vi "MyG#G3SubTempl_GetAttributesToModify.vi"(0 "reference in":refnum<class "MyG#G3SubTempl.lvclass">, 3 "timeout in ms (-1)":i32=-1, 5 "error in (no error)":errorcluster) -> (14 "reference out":refnum<class "MyG#G3SubTempl.lvclass">, 15 "attributes ref":T3, 16 "attributes":T1, 17 "timeout":bool, 19 "error out":errorcluster)   [LabVIEW 2020, in "MyG#G3SubTempl.lvclass"]
doc: "This VI returns the class attributes associated with the object reference and places a lock on the object. If reference is wired, the class attributes of this class (or sub class) will be returned else the class attributes will default to the class.\n\nIf the object is currently locked for modification by another method, 'Timeout' specifies how long the VI should wait to receive access to the object. The default value waits until the object becomes available.\n\nYou must use this class SetModifiedClassAttributes VI to set the object's data and release the lock."
uses:
  MyG#G3SubTempl.lvclass
  C:/Program Files (x86)/National Instruments/LabVIEW 2020/examples/AddQ/G#/CreateDestroy/MyG#G3Templ_class/MyG#G3Templ.lvclass
  ObjectAttributesRef.ctl
  protected/ObjectAttributes.ctl
  MyG#G3Templ_class/protected/ObjectAttributes.ctl
  MyG#G3SubTempl.lvclass/MyG#G3SubTempl.ctl
  MyG#G3Templ_class/MyG#G3Templ.lvclass
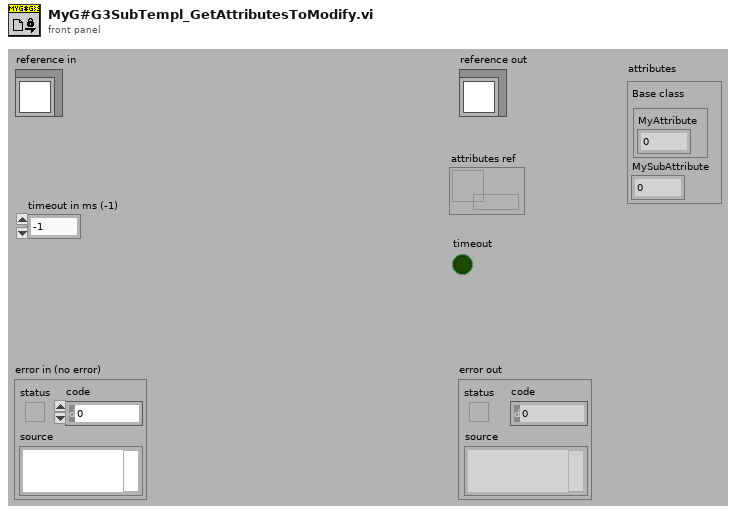
[diagram p1: front panel]
types:
  T1 = typedef "MyG#G3SubTempl.lvclass/ObjectAttributes.ctl" = cluster{"Base class":T2, "MySubAttribute":dbl}
  T2 = typedef "MyG#G3Templ.lvclass/ObjectAttributes.ctl" = cluster{"MyAttribute":dbl}
  T3 = typedef "MyG#G3SubTempl.lvclass/ObjectAttributesRef.ctl" = refnum<data-value>
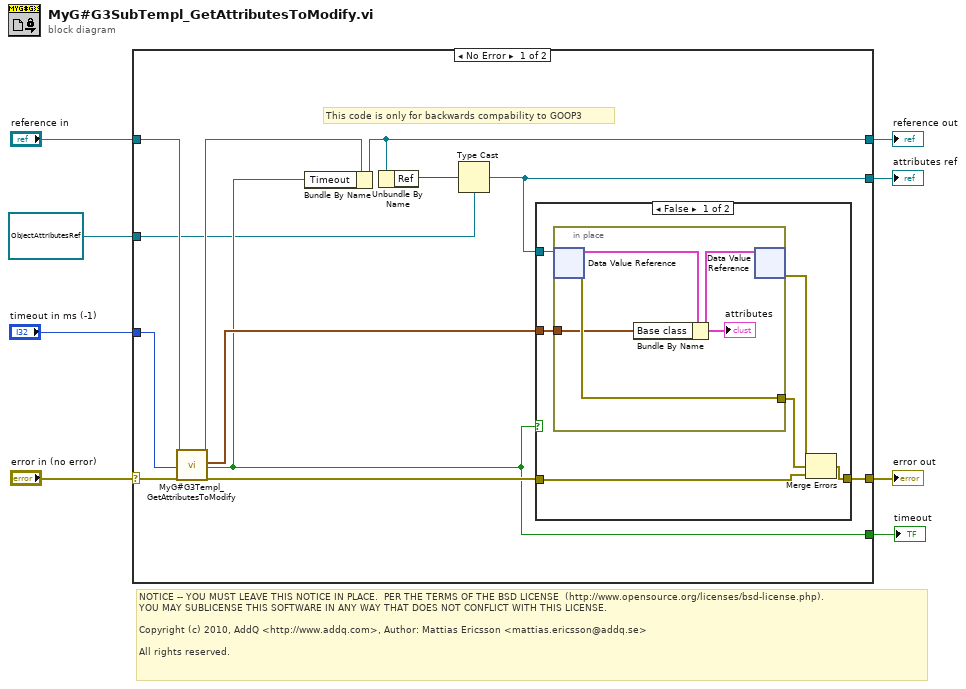
[diagram p0: block diagram]
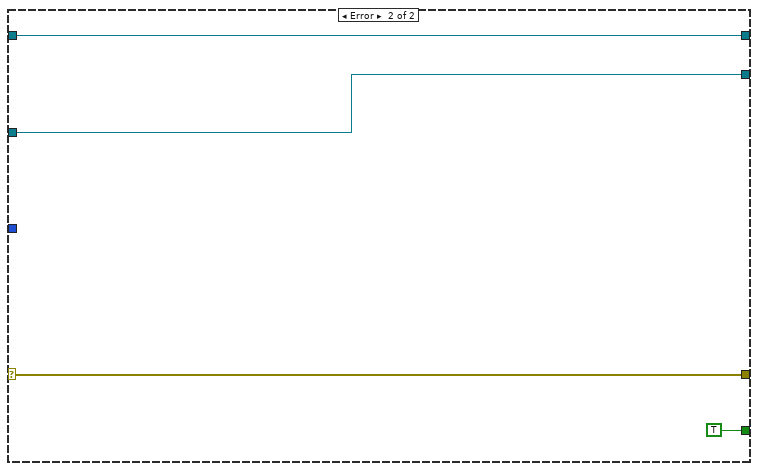
[diagram p3: hidden frame]
diagram:
  # "NOTICE -- YOU MUST LEAVE THIS NOTICE IN PLACE.  PER THE TERMS OF THE BSD LICENSE  (http://www.opensource.org/licenses/bsd-license.php).\nYOU MAY SUBLICENSE THIS SOFTWARE IN ANY WAY THAT DOES NOT CONFLICT WITH THIS LICENSE.\n\nCopyright (c) 2010, AddQ <http://www.addq.com>, Author: Mattias Ericsson <mattias.ericsson@addq.se>\n\nAll rights reserved."
  n1 = case shown="No Error" "error in (no error)" {
    selector: "error in (no error)" -> [w19 w35]
    tunnel: [w20 w35] -> w7
    tunnel: [w15 w34] -> w5
    tunnel: "reference in" -> [w13 w34]
    tunnel: [w10 w32] -> w4
    tunnel: "timeout in ms (-1)" -> [w18 _]
    tunnel: [w14 TRUE ("status")] -> w2
    tunnel: T3 refnum ("attributes ref") -> [w9 w32]
    frame No Error {
      # "This code is only for backwards compability to GOOP3"
      n2 = call "MyG#G3Templ_GetAttributesToModify.vi"("reference in"=w13, "timeout in ms (-1)"=w18, "error in (no error)"=w19) -> ("reference out"=w12:refnum<class "MyG#G3SubTempl.lvclass">, "attributes"=w16:T2, "timeout"=w14:bool, "error out"=w17:errorcluster)  [unwired: 12 in, 1 out]
      n3 = Bundle By Name(cluster=w12, "Timeout"=w14) -> (w15:refnum<class "MyG#G3SubTempl.lvclass">)
      n4 = Unbundle By Name(w15) -> ("Ref"=w11:u32)
      n5 = Type Cast(type=w9, x=w11) -> (*(type *) &x=w10:T3)
      n6 = case shown="False" w14 {
        tunnel: w10 -> [w26 _]
        tunnel: w17 -> [w25 w31]
        tunnel: [w22 w31] -> w20
        tunnel: w16 -> [w21 _]
        frame False {
          n7 = in-place {
            in-place-border: [w28] -> w24
            in-place-border: w21 -> [w27]
            n8 = in-place-dvr #1(w26) -> (w30:T1, w28:errorcluster)
            n9 = Bundle By Name(cluster=w30, "Base class"=w27) -> (w29:T1)
            "attributes" <- w29
            n10 = in-place-dvr #1(w29) -> (w23:errorcluster)  [unwired: 1 out]
          }
          n11 = Merge Errors(w23, w24, w25) -> (w22:errorcluster)
        }
        frame True {
        }
      }
    }
    frame Error {
    }
  }
  "error out" <- w7
  "reference out" <- w5
  "attributes ref" <- w4
  "timeout" <- w2
